vi "GCodeIntegrityTest.vi"() -> ()   [LabVIEW 2017]
panel:
  out "Failed Test Cases":T1(array[cluster])
  out "Files Processed":dbl
  out "Test Cases":T1(array[cluster])
  out "All Files Found":bool
  out "Report":string
  out "error out":errorcluster
  in  "error in":errorcluster
  in  "Source VI(s)":path=path ""
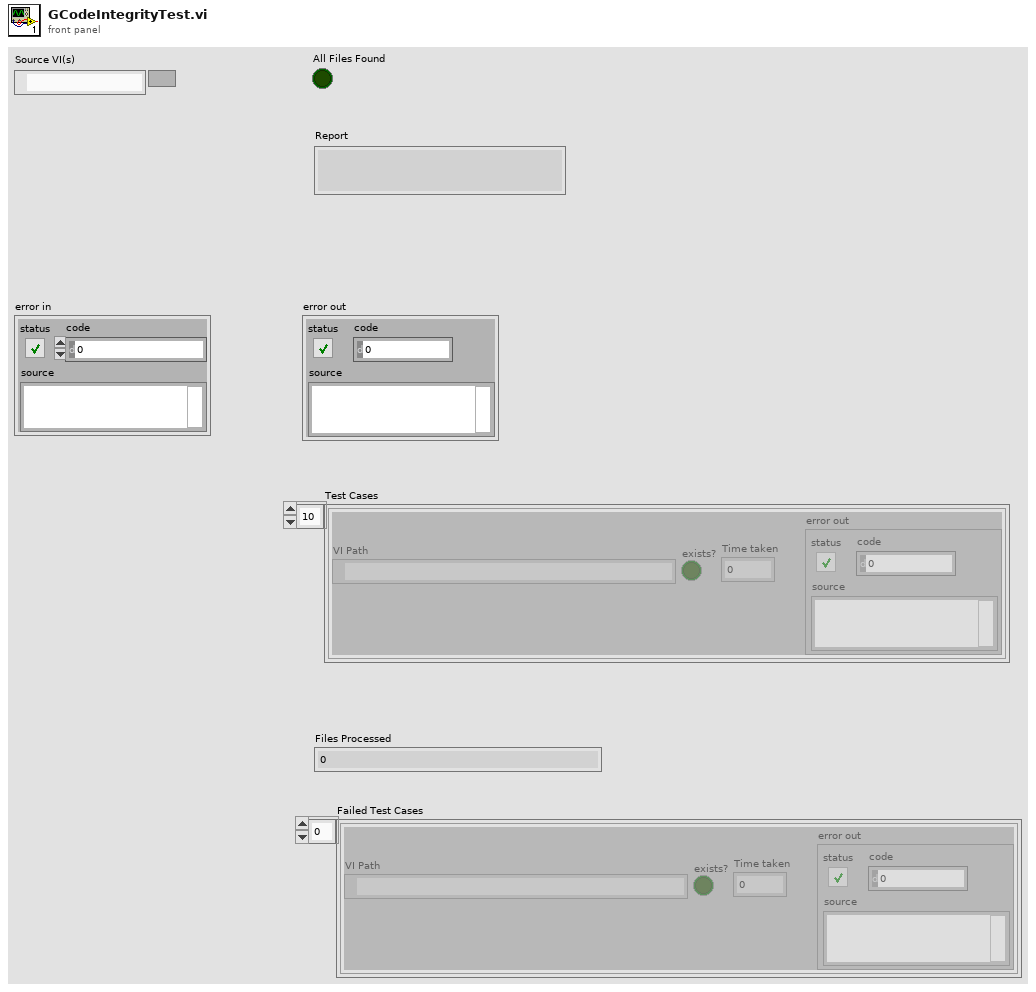
[diagram p1: front panel]
types:
  T1 = cluster{"VI Path":path, "exists?":bool, "Time taken":dbl, "error out":errorcluster}[]
  T2 = cluster{"VI Path":path, "exists?":bool, "Time taken":dbl, "error out":errorcluster}
  T3 = enum16{"open", "open or create", "create or replace", "create", "open (read only)"}
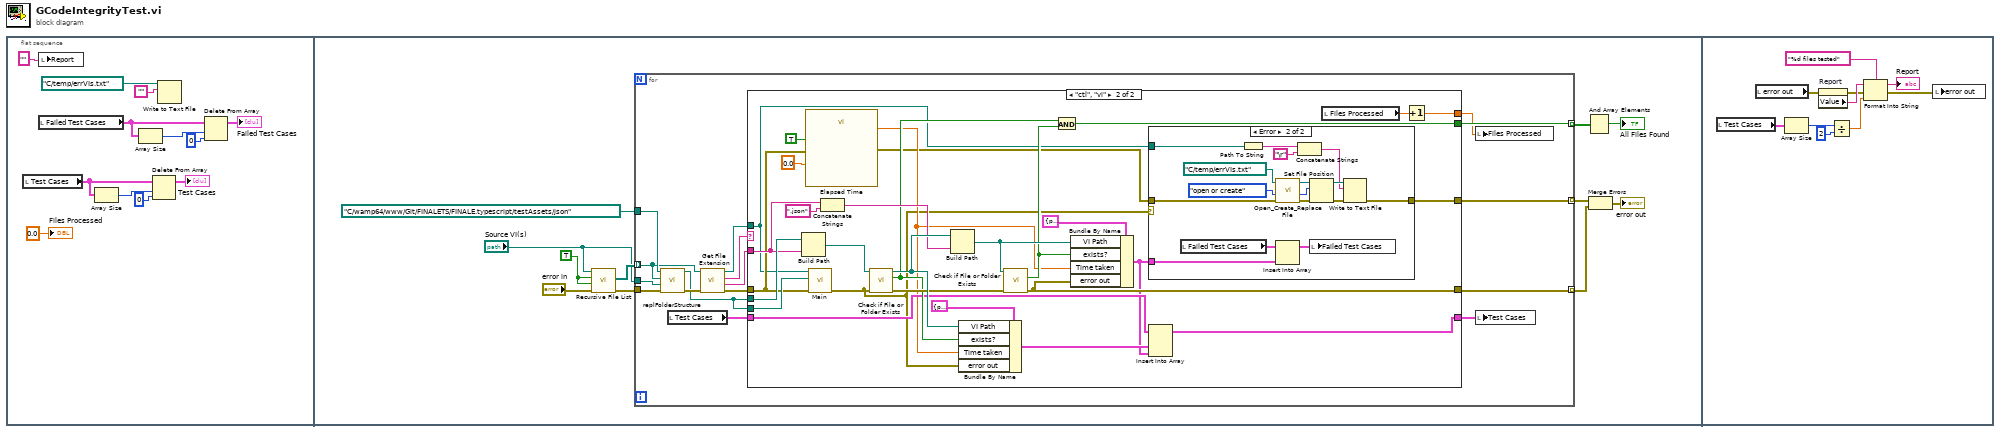
[diagram p0: block diagram]
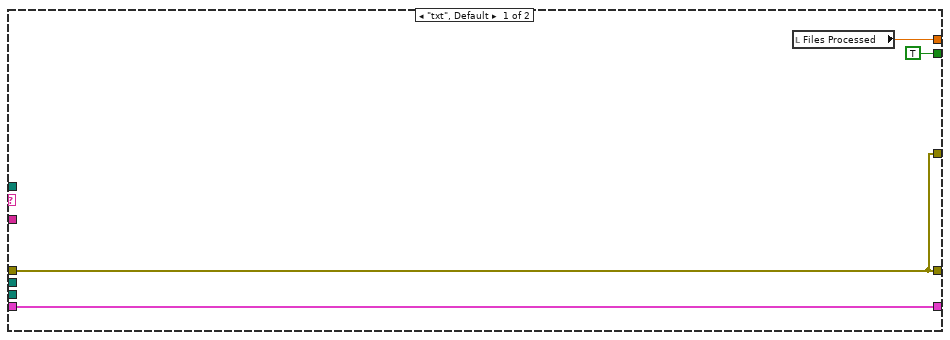
[diagram p2: hidden frame]
diagram:
  n1 = flat-sequence {
    frame #0 {
      n2 = local read "Test Cases"() -> (w11:T1)
      n3 = local read "Failed Test Cases"() -> (w5:T1)
      n4 = local write "Report"("" ("Report")) -> ()
      n5 = Array Size(array=w11) -> (size(s)=w10:i32)
      n6 = Array Size(array=w5) -> (size(s)=w6:i32)
      n7 = Delete From Array(array=w11, length=w10, index=0) -> (array with subset deleted=→"Test Cases":T1)  [unwired: 1 out]
      n8 = Write to Text File(file (use dialog)=path "C:/temp/errVIs.txt" ("file path"), text="") -> ()  [unwired: 2 in, 3 out]
      n9 = Delete From Array(array=w5, length=w6, index=0) -> (array with subset deleted=→"Failed Test Cases":T1)  [unwired: 1 out]
      "Files Processed" <- 0.0 ("Files Processed")
    }
    frame #1 {
      w23 = TRUE ("Treat LLBs as Folders?")
      n10 = call <vilib>:"Recursive File List.vi"("error in (no error)"="error in", "Continue Recursing on Error? (F)"=w23, "Treat LLBs as Folders?"=w23, "Folder Path"="Source VI(s)") -> ("error out"=w21:errorcluster, "All Files in Dir"=w20:path[])  [unwired: 3 in, 3 out]
      n11 = for {
        tunnel: w21 -> [w35]
        tunnel: w20 -> [w32] mode=indexing
        tunnel: path "C:/wamp64/www/Git/FINALETS/FINALE.typescript/testAssets/json" ("Destination Directory") -> [w33]
        tunnel: "Source VI(s)" -> [w36]
        tunnel: [w28] -> w17 mode=indexing
        tunnel: [w27] -> w15 mode=indexing
        tunnel: [w26] -> w13 mode=indexing
        n12 = call "replFolderStructure.vi"("error in (no error)"=w35, "VI origin folder"=w36, "file path"=w32, "Destination Directory"=w33) -> ("error out"=w34:errorcluster, "dup path"=w25:path)  [unwired: 6 in]
        n13 = local read "Test Cases"() -> (w30:T1)
        n14 = call <vilib>:"Get File Extension.vi"("error in (no error)"=w34, "file"=w32) -> ("error out"=w38:errorcluster, "filename without extension"=w37:string, "lowercase file extension"=w39:string, "dup file"=w31:path)  [unwired: 5 in, 1 out]
        n15 = case shown="\"ctl\", \"vi\"" w39 {
          tunnel: [w41 w48] -> w27
          tunnel: w25 -> [_ w64]
          tunnel: w38 -> [w41 w57]
          tunnel: w37 -> [_ w62]
          tunnel: [w42 w67] -> w29
          tunnel: [TRUE w51] -> w28
          tunnel: w25 -> [_ w61]
          tunnel: w31 -> [_ w50]
          tunnel: w30 -> [w42 w60]
          tunnel: [w41 w53] -> w26
          tunnel: [w40 w46] -> w24
          frame "txt", Default {
            n16 = local read "Files Processed"() -> (w40:dbl)
          }
          frame "ctl", "vi" {
            n17 = Build Path(base path=w64, name or relative path=w62) -> (appended path=w63:path)
            n18 = call "Elapsed Time"("Auto Reset"=TRUE, "error in (no error)"=w57, "Set Start Time (s)"=0.0) -> ("Elapsed Time (s)"=w56:dbl, "error out"=w49:errorcluster)  [unwired: 9 in, 6 out]
            n19 = call "Main.vi"("error in"=w57, "Destination Directory"=w61, "Source VI(s)"=w50) -> ("error out"=w44:errorcluster)  [unwired: 8 in]
            n20 = Concatenate Strings(w62, ".json" ("string")) -> (w70:string)
            n21 = call <vilib>:"Check if File or Folder Exists.vi"("error in (no error)"=w44, "path"=w63) -> ("error out"=w69:errorcluster, "file or folder exists?"=w66:bool, "dup path"=w72:path)  [unwired: 7 in]
            n22 = Build Path(base path=w72, name or relative path=w70) -> (appended path=w68:path)
            n23 = Bundle By Name(cluster=T2 {"VI Path"=path "C:/wamp64/www/Git/FINALETS/FINALE.typescript/testAssets/json/Event_Structures", "exists?"=TRUE, "Time taken"=0.0, "error out"={"status"=FALSE, "code"=0, "source"=""}}, "VI Path"=w72, "exists?"=w66, "Time taken"=w56, "error out"=w44) -> (w59:T2)
            n24 = call <vilib>:"Check if File or Folder Exists.vi"("error in (no error)"=w69, "path"=w68) -> ("error out"=w53:errorcluster, "file or folder exists?"=w65:bool)  [unwired: 7 in, 1 out]
            n25 = And(x=w66, y=w65) -> (x .and. y?=w51:bool)
            n26 = Bundle By Name(cluster=T2 {"VI Path"=path "C:/wamp64/www/Git/FINALETS/FINALE.typescript/testAssets/json/Event_Structures", "exists?"=TRUE, "Time taken"=0.0, "error out"={"status"=FALSE, "code"=0, "source"=""}}, "VI Path"=w68, "exists?"=w65, "Time taken"=w56, "error out"=w53) -> (w45:T2)
            n27 = case shown="Error" w44 {
              tunnel: w50 -> [_ w81]
              tunnel: w49 -> [w73 w87]
              tunnel: [w73 w80] -> w48
              tunnel: w45 -> [_ w79]
              frame No Error {
              }
              frame Error {
                n28 = local read "Failed Test Cases"() -> (w78:T1)
                n29 = Path To String(path=w81) -> (string=w76:string)
                n30 = call <vilib>:"Open_Create_Replace File.vi"("error in (no error)"=w87, "function (open:0)"=T3."open or create", "file path"=path "C:/temp/errVIs.txt") -> ("error out"=w84:errorcluster, "file size (bytes)"=w85:i32, "refnum"=w86:refnum<file>)  [unwired: 5 in, 1 out]
                n31 = Insert Into Array(array=w78, new element=w79) -> (w77:T1)  [unwired: 1 in]
                n32 = Concatenate Strings(w76, "\r") -> (w75:string)
                n33 = Set File Position(offset (in bytes) (0)=w85, refnum=w86, error in=w84) -> (refnum out=w82:refnum<file>, error out=w83:errorcluster)  [unwired: 1 in]
                n34 = local write "Failed Test Cases"(w77) -> ()
                n35 = Write to Text File(file (use dialog)=w82, text=w75, error in=w83) -> (error out=w80:errorcluster)  [unwired: 1 in, 2 out]
              }
            }
            n36 = Insert Into Array(array=w60, new element #1=w59, new element #2=w45) -> (w67:T1)  [unwired: 1 in]
            n37 = local read "Files Processed"() -> (w47:dbl)
            n38 = Increment(x=w47) -> (x+1=w46:dbl)
          }
        }
        n39 = local write "Files Processed"(w24) -> ()
        n40 = local write "Test Cases"(w29) -> ()
      }
      n41 = And Array Elements(Boolean array=w17) -> (logical AND=→"All Files Found":bool)
      n42 = Merge Errors(w15, w13) -> (→"error out":errorcluster)
    }
    frame #2 {
      n43 = local read "Test Cases"() -> (w99:T1)
      n44 = local read "error out"() -> (w95:errorcluster)
      n45 = Array Size(array=w99) -> (size(s)=w92:i32)
      n46 = property on="Report" class="Str"(error in=w95) -> (error out=w94:errorcluster, "Value"=w96:string)  [unwired: 1 in, 1 out]
      n47 = Divide(x=w92, y=2) -> (x/y=w90:dbl)
      n48 = Format Into String(format string="%d files tested", initial string=w96, error in=w94, w90) -> (resulting string=→"Report":string, error out=w97:errorcluster)
      n49 = local write "error out"(w97) -> ()
    }
  }
